vi "Efficiency Plot.vi"(0 "SMU 1 (Source)":refnum<k15>="4139_1", 1 "Voltage Steps":dbl[](array[numeric])=[8.5, 12.0, 24.0, 36.0, 48.0, 60.0], 5 "SMU 2 (Sink)":refnum<k15>="4139_2", 7 "Current Sweep Start":dbl format="%0.2f", 9 "Current Sweep End":dbl=-3.0 format="%0.2f", 11 "Error In":errorcluster, 12 "# Points":i32=50) -> (6 "Efficiency Plot":cluster{"current measurements":dbl[], dbl[]}[](graph)=[{"current measurements"=[0.0, 0.061224489795918366, 0.12244897959183673, 0.1836734693877551, 0.24489795918367346, 0.30612244897959184, 0.3673469387755102, 0.42857142857142855, 0.4897959183673469, 0.5510204081632653, 0.6122448979591837, 0.673469387755102, 0.7346938775510204, 0.7959183673469388, 0.8571428571428571, 0.9183673469387755, 0.9795918367346939, 1.0408163265306123, 1.1020408163265305, 1.163265306122449, 1.2244897959183674, 1.2857142857142858, 1.346938775510204, 1.4081632653061225, 1.469387755102041, 1.530612244897959, 1.5918367346938775, 1.653061224489796, 1.7142857142857142, 1.7755102040816326, 1.836734693877551, 1.8979591836734695, 1.9591836734693877, 2.020408163265306, 2.0816326530612246, 2.142857142857143, 2.204081632653061, 2.2653061224489797, 2.326530612244898, 2.3877551020408165, 2.4489795918367347, 2.510204081632653, 2.5714285714285716, 2.63265306122449, 2.693877551020408, 2.7551020408163267, 2.816326530612245, 2.877551020408163, 2.938775510204082, 3.0], [nan, inf, inf, inf, inf, inf, inf, inf, inf, inf, inf, inf, inf, inf, inf, inf, inf, inf, inf, inf, inf, inf, inf, inf, inf, inf, inf, inf, inf, inf, inf, inf, inf, inf, inf, inf, inf, inf, inf, inf, inf, inf, inf, inf, inf, inf, inf, inf, inf, inf]}, {"current measurements"=[0.0, 0.061224489795918366, 0.12244897959183673, 0.1836734693877551, 0.24489795918367346, 0.30612244897959184, 0.3673469387755102, 0.42857142857142855, 0.4897959183673469, 0.5510204081632653, 0.6122448979591837, 0.673469387755102, 0.7346938775510204, 0.7959183673469388, 0.8571428571428571, 0.9183673469387755, 0.9795918367346939, 1.0408163265306123, 1.1020408163265305, 1.163265306122449, 1.2244897959183674, 1.2857142857142858, 1.346938775510204, 1.4081632653061225, 1.469387755102041, 1.530612244897959, 1.5918367346938775, 1.653061224489796, 1.7142857142857142, 1.7755102040816326, 1.836734693877551, 1.8979591836734695, 1.9591836734693877, 2.020408163265306, 2.0816326530612246, 2.142857142857143, 2.204081632653061, 2.2653061224489797, 2.326530612244898, 2.3877551020408165, 2.4489795918367347, 2.510204081632653, 2.5714285714285716, 2.63265306122449, 2.693877551020408, 2.7551020408163267, 2.816326530612245, 2.877551020408163, 2.938775510204082, 3.0], [nan, inf, inf, inf, inf, inf, inf, inf, inf, inf, inf, inf, inf, inf, inf, inf, inf, inf, inf, inf, inf, inf, inf, inf, inf, inf, inf, inf, inf, inf, inf, inf, inf, inf, inf, inf, inf, inf, inf, inf, inf, inf, inf, inf, inf, inf, inf, inf, inf, inf]}, {"current measurements"=[0.0, 0.061224489795918366, 0.12244897959183673, 0.1836734693877551, 0.24489795918367346, 0.30612244897959184, 0.3673469387755102, 0.42857142857142855, 0.4897959183673469, 0.5510204081632653, 0.6122448979591837, 0.673469387755102, 0.7346938775510204, 0.7959183673469388, 0.8571428571428571, 0.9183673469387755, 0.9795918367346939, 1.0408163265306123, 1.1020408163265305, 1.163265306122449, 1.2244897959183674, 1.2857142857142858, 1.346938775510204, 1.4081632653061225, 1.469387755102041, 1.530612244897959, 1.5918367346938775, 1.653061224489796, 1.7142857142857142, 1.7755102040816326, 1.836734693877551, 1.8979591836734695, 1.9591836734693877, 2.020408163265306, 2.0816326530612246, 2.142857142857143, 2.204081632653061, 2.2653061224489797, 2.326530612244898, 2.3877551020408165, 2.4489795918367347, 2.510204081632653, 2.5714285714285716, 2.63265306122449, 2.693877551020408, 2.7551020408163267, 2.816326530612245, 2.877551020408163, 2.938775510204082, 3.0], [nan, inf, inf, inf, inf, inf, inf, inf, inf, inf, inf, inf, inf, inf, inf, inf, inf, inf, inf, inf, inf, inf, inf, inf, inf, inf, inf, inf, inf, inf, inf, inf, inf, inf, inf, inf, inf, inf, inf, inf, inf, inf, inf, inf, inf, inf, inf, inf, inf, inf]}, {"current measurements"=[0.0, 0.061224489795918366, 0.12244897959183673, 0.1836734693877551, 0.24489795918367346, 0.30612244897959184, 0.3673469387755102, 0.42857142857142855, 0.4897959183673469, 0.5510204081632653, 0.6122448979591837, 0.673469387755102, 0.7346938775510204, 0.7959183673469388, 0.8571428571428571, 0.9183673469387755, 0.9795918367346939, 1.0408163265306123, 1.1020408163265305, 1.163265306122449, 1.2244897959183674, 1.2857142857142858, 1.346938775510204, 1.4081632653061225, 1.469387755102041, 1.530612244897959, 1.5918367346938775, 1.653061224489796, 1.7142857142857142, 1.7755102040816326, 1.836734693877551, 1.8979591836734695, 1.9591836734693877, 2.020408163265306, 2.0816326530612246, 2.142857142857143, 2.204081632653061, 2.2653061224489797, 2.326530612244898, 2.3877551020408165, 2.4489795918367347, 2.510204081632653, 2.5714285714285716, 2.63265306122449, 2.693877551020408, 2.7551020408163267, 2.816326530612245, 2.877551020408163, 2.938775510204082, 3.0], [nan, inf, inf, inf, inf, inf, inf, inf, inf, inf, inf, inf, inf, inf, inf, inf, inf, inf, inf, inf, inf, inf, inf, inf, inf, inf, inf, inf, inf, inf, inf, inf, inf, inf, inf, inf, inf, inf, inf, inf, inf, inf, inf, inf, inf, inf, inf, inf, inf, inf]}, {"current measurements"=[0.0, 0.061224489795918366, 0.12244897959183673, 0.1836734693877551, 0.24489795918367346, 0.30612244897959184, 0.3673469387755102, 0.42857142857142855, 0.4897959183673469, 0.5510204081632653, 0.6122448979591837, 0.673469387755102, 0.7346938775510204, 0.7959183673469388, 0.8571428571428571, 0.9183673469387755, 0.9795918367346939, 1.0408163265306123, 1.1020408163265305, 1.163265306122449, 1.2244897959183674, 1.2857142857142858, 1.346938775510204, 1.4081632653061225, 1.469387755102041, 1.530612244897959, 1.5918367346938775, 1.653061224489796, 1.7142857142857142, 1.7755102040816326, 1.836734693877551, 1.8979591836734695, 1.9591836734693877, 2.020408163265306, 2.0816326530612246, 2.142857142857143, 2.204081632653061, 2.2653061224489797, 2.326530612244898, 2.3877551020408165, 2.4489795918367347, 2.510204081632653, 2.5714285714285716, 2.63265306122449, 2.693877551020408, 2.7551020408163267, 2.816326530612245, 2.877551020408163, 2.938775510204082, 3.0], [nan, inf, inf, inf, inf, inf, inf, inf, inf, inf, inf, inf, inf, inf, inf, inf, inf, inf, inf, inf, inf, inf, inf, inf, inf, inf, inf, inf, inf, inf, inf, inf, inf, inf, inf, inf, inf, inf, inf, inf, inf, inf, inf, inf, inf, inf, inf, inf, inf, inf]}, {"current measurements"=[0.0, 0.061224489795918366, 0.12244897959183673, 0.1836734693877551, 0.24489795918367346, 0.30612244897959184, 0.3673469387755102, 0.42857142857142855, 0.4897959183673469, 0.5510204081632653, 0.6122448979591837, 0.673469387755102, 0.7346938775510204, 0.7959183673469388, 0.8571428571428571, 0.9183673469387755, 0.9795918367346939, 1.0408163265306123, 1.1020408163265305, 1.163265306122449, 1.2244897959183674, 1.2857142857142858, 1.346938775510204, 1.4081632653061225, 1.469387755102041, 1.530612244897959, 1.5918367346938775, 1.653061224489796, 1.7142857142857142, 1.7755102040816326, 1.836734693877551, 1.8979591836734695, 1.9591836734693877, 2.020408163265306, 2.0816326530612246, 2.142857142857143, 2.204081632653061, 2.2653061224489797, 2.326530612244898, 2.3877551020408165, 2.4489795918367347, 2.510204081632653, 2.5714285714285716, 2.63265306122449, 2.693877551020408, 2.7551020408163267, 2.816326530612245, 2.877551020408163, 2.938775510204082, 3.0], [nan, inf, inf, inf, inf, inf, inf, inf, inf, inf, inf, inf, inf, inf, inf, inf, inf, inf, inf, inf, inf, inf, inf, inf, inf, inf, inf, inf, inf, inf, inf, inf, inf, inf, inf, inf, inf, inf, inf, inf, inf, inf, inf, inf, inf, inf, inf, inf, inf, inf]}], 15 "Error Out":errorcluster)   [LabVIEW 2014]
doc: "Demonstrates how to use triggers and events to synchronize multiple channels in Sequence source mode. Use this example to sequence multiple channels in lock-step."
uses:
  <instrlib>/niDCPower/nidcpower.llb/niDCPower Output Function.ctl
  <instrlib>/niDCPower/nidcpower.llb/niDCPower Source Mode.ctl
  <instrlib>/niDCPower/nidcpower.llb/niDCPower Sense.ctl
  <instrlib>/niDCPower/nidcpower.llb/niDCPower Sequence Attribute Type.ctl
  <instrlib>/niDCPower/nidcpower.llb/niDCPower Disable Source Trigger.vi
  <instrlib>/niDCPower/nidcpower.llb/niDCPower Configure Digital Edge Source Trigger.vi
  <instrlib>/niDCPower/nidcpower.llb/niDCPower Configure Digital Edge Measure Trigger.vi
panel:
  # "Sink"
  # "SOURCING OPERATION (SMU 1)\n1. Source Voltage Level and Fire Source Trigger Event \n2. Wait \"Delay\" Seconds\n3. Fire Source Complete Event\n3. Measure Current Immediately\n\nIV1, IV2, IV3...IV300 at V IN"
  # "SINKING OPERATION (SMU 2)\n1. Source Current Level (SMU1 Trigger)\n2. Wait \"Delay\" Seconds\n3. Measure Voltage (Using SMU1 Source Complete Event Trigger)\n\n\nIV1, IV2, IV3...IV300 at V OUT"
  # "Source"
  # "Iout = 0 to 3 A"
  # "Vin = 8 to 60 V"
  # "Vout = 5 V"
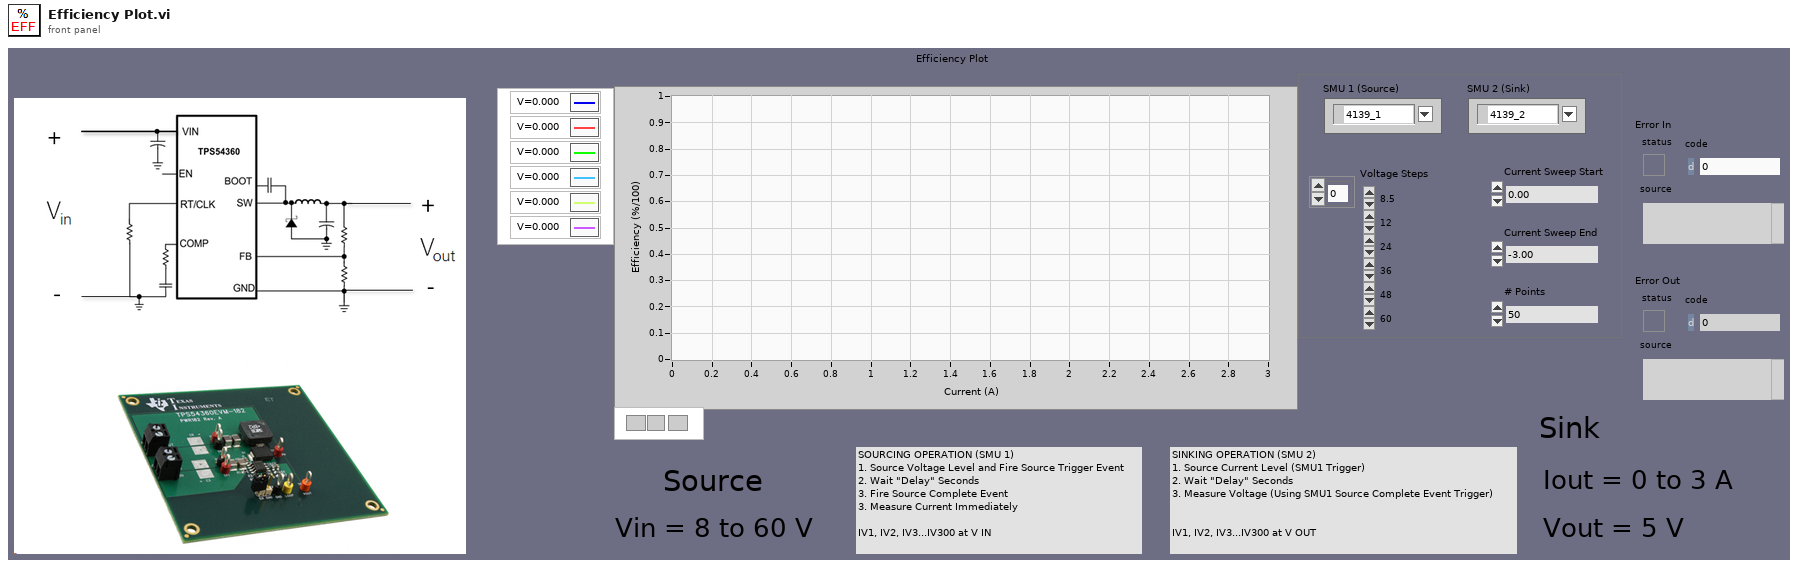
[diagram p1: front panel]
types:
  T1 = typedef "niDCPower Sequence Attribute Type.ctl" = i32
  T2 = typedef "niDCPower Sense.ctl" = i32
  T3 = typedef "niDCPower Source Mode.ctl" = i32
  T4 = typedef "niDCPower Output Function.ctl" = i32
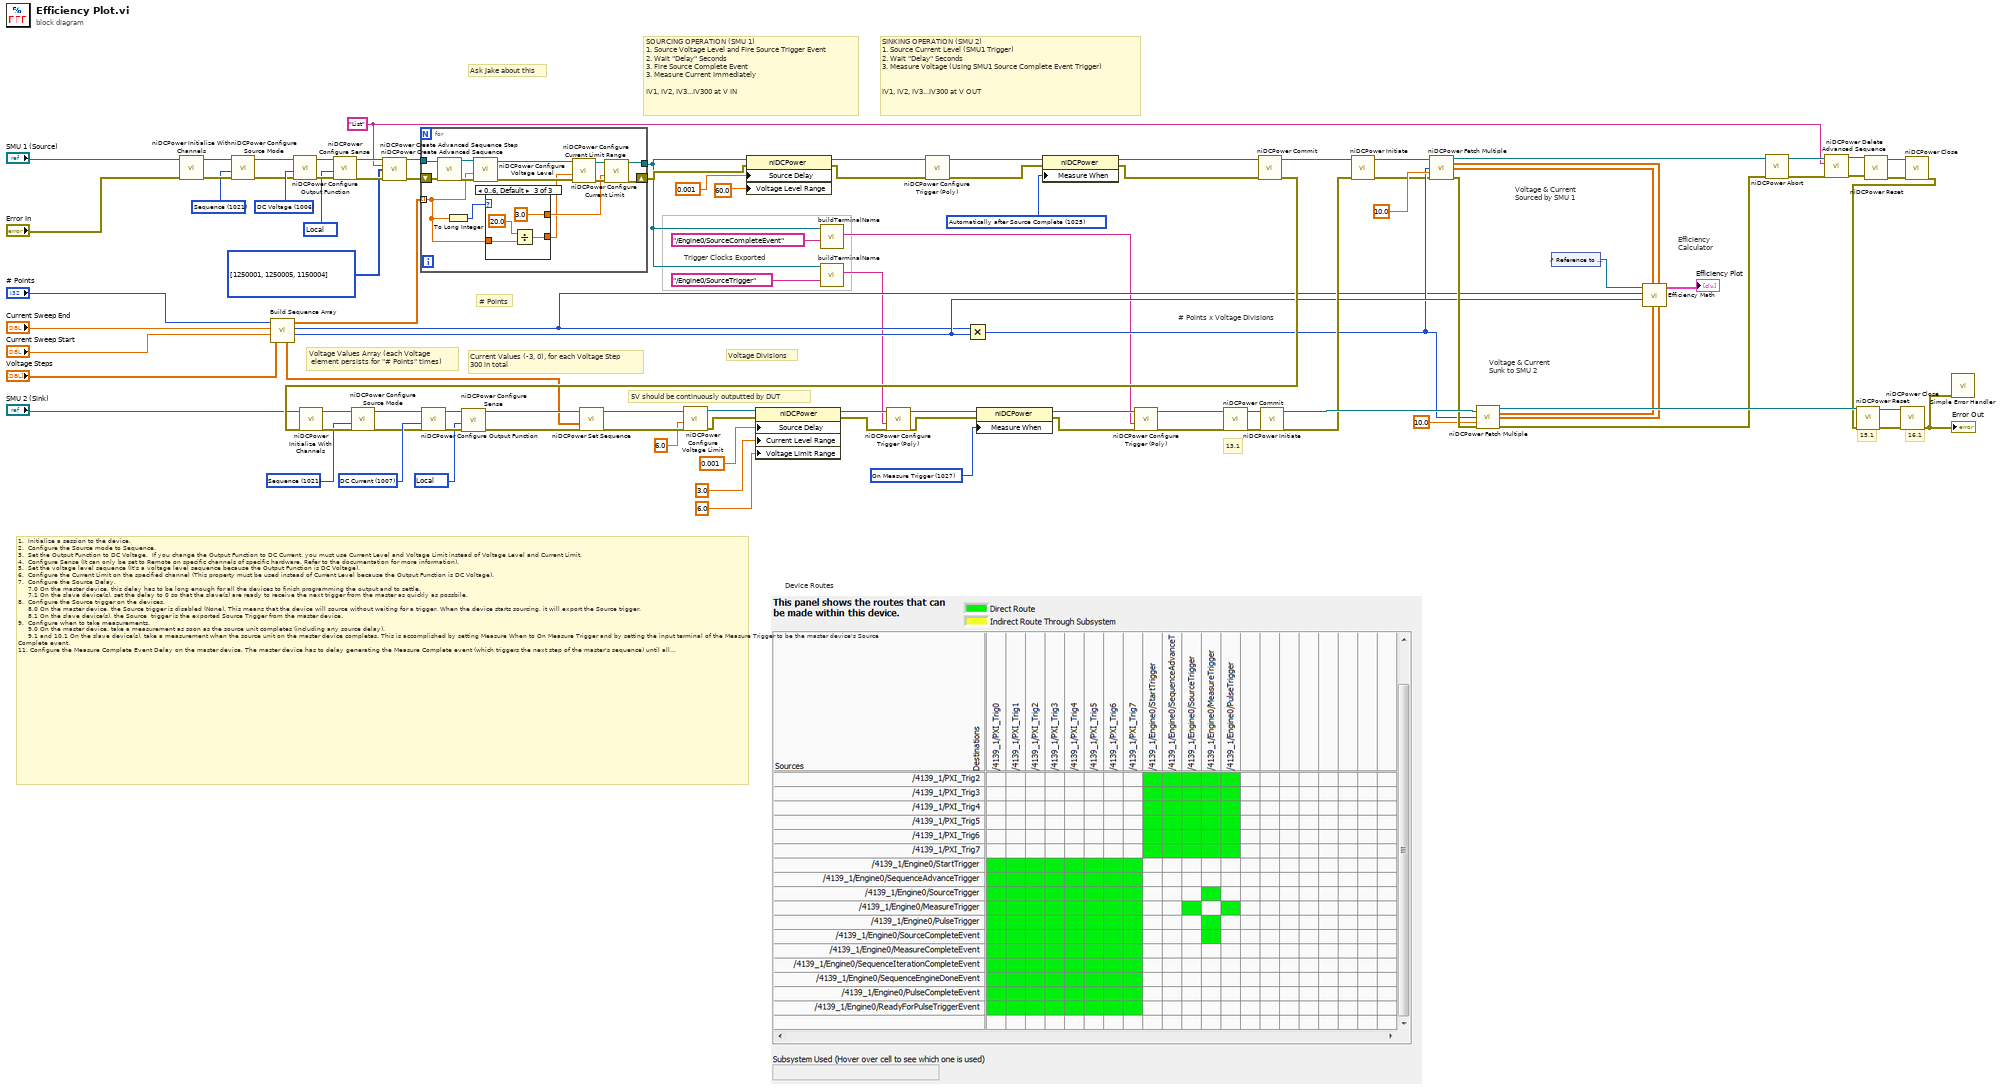
[diagram p0: block diagram]
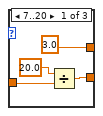
[diagram p2: hidden frame]
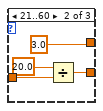
[diagram p3: hidden frame]
diagram:
  w2 = "List" ("list name")
  w18 = T1[] [1250001, 1250005, 1150004] items=["Voltage Pole-Zero Ratio"=1150069, "Voltage Compensation Frequency"=1150068, "Voltage Gain Bandwidth"=1150067, "Transient Response"=1150062, "Output Resistance"=1150061, "Output Connected"=1150060, "Output Enabled"=1250006, "Output Function"=1150008, "Source Delay"=1150051, "Aperture Time Units"=1150059, "Aperture Time"=1150058, "Voltage Limit Range"=1150012, "Voltage Limit"=1150010, "Current Level Range"=1150011, "Current Level"=1150009, "Current Limit Range"=1150004, "Current Limit"=1250005, "Voltage Level Range"=1150005, "Voltage Level"=1250001]
  w52 = T2 1008 items=["Local"=1008, "Remote"=1009] ("sense")
  w53 = T2 1008 items=["Local"=1008, "Remote"=1009] ("sense")
  w65 = 1027 items=["Automatically after Source Complete"=1025, "On Demand"=1026, "On Measure Trigger"=1027] ("Measurement:Advanced:Measure When")
  w66 = T3 1021 items=["Single Point"=1020, "Sequence"=1021] ("source mode")
  w77 = T4 1007 items=["DC Voltage"=1006, "DC Current"=1007] ("output function")
  w86 = 1025 items=["Automatically after Source Complete"=1025, "On Demand"=1026, "On Measure Trigger"=1027] ("Measurement:Advanced:Measure When")
  w87 = T3 1021 items=["Single Point"=1020, "Sequence"=1021] ("source mode")
  w94 = T4 1006 items=["DC Voltage"=1006, "DC Current"=1007] ("output function")
  # "Trigger Clocks Exported"
  # "Device Routes"
  # "Efficiency\nCalculator"
  # "Voltage & Current \nSourced by SMU 1"
  # "Voltage & Current \nSunk to SMU 2"
  # "# Points x Voltage Divisions"
  # "Ask Jake about this"
  # "SINKING OPERATION (SMU 2)\n1. Source Current Level (SMU1 Trigger)\n2. Wait \"Delay\" Seconds\n3. Measure Voltage (Using SMU1 Source Complete Event Trigger)\n\n\nIV1, IV2, IV3...IV300 at V OUT"
  # "SOURCING OPERATION (SMU 1)\n1. Source Voltage Level and Fire Source Trigger Event \n2. Wait \"Delay\" Seconds\n3. Fire Source Complete Event\n3. Measure Current Immediately\n\nIV1, IV2, IV3...IV300 at V IN"
  # "Voltage Divisions"
  # "# Points"
  # "5V should be continuously outputted by DUT"
  # "Voltage Values Array (each Voltage\n element persists for \"# Points\" times)"
  # "Current Values (-3, 0), for each Voltage Step\n300 in total"
  # "16.1"
  # "15.1"
  # "13.1"
  # "1.  Initialize a session to the device.\n2.  Configure the Source mode to Sequence.\n3.  Set the Output Function to DC Voltage.  If you change the Output Function to DC Current, you must use Current Level and Voltage Limit instead of Voltage Level and Current Limit.\n4.  Configure Sense (It can only be set to Remote on specific channels of specific hardware. Refer to the documentation for more information).\n5.  Set the voltage level sequence (It's a voltage level sequence because the Output Function is DC Voltage).\n6.  Configure the Current Limit on the specified channel (This property must be used instead of Current Level because the Output Function is DC Voltage).\n7.  Configure the Source Delay.\n     7.0 On the master device, this delay has to be long enough for all the devices to finish programming the output and to settle.\n     7.1 On the slave device(s), set the delay to 0 so that the slave(s) are ready to receive the next trigger from the master as quickly as possbile.\n8.  Configure the Source trigger on the devices.\n     8.0 On the master device, the Source trigger is disabled (None). This means that the device will source without waiting for a trigger. When the device starts sourcing, it will export the Source trigger.\n     8.1 On the slave device(s), the Source  trigger is the exported Source Trigger from the master device.\n9.  Configure when to take measurements.\n     9.0 On the master device, take a measurement as soon as the source unit completes (including any source delay).\n     9.1 and 10.1 On the slave device(s), take a measurement when the source unit on the master device completes. This is accomplished by setting Measure When to On Measure Trigger and by setting the input terminal of the Measure Trigger to be the master device's Source Complete event.\n11. Configure the Measure Complete Event Delay on the master device. The master device has to delay generating the Measure Complete event (which triggers the next step of the master's sequence) until all slave device(s) have completed taking measurements. The amount of time a slave takes to measure can vary based on its configuration and model.\n12. Commit the settings to the device so that the driver establishes all the routing required for the configured triggers and events."
  n1 = call <instrlib>:"niDCPower Initialize With Channels.vi"("error in (no error)"="Error In", "resource name"="SMU 1 (Source)") -> ("error out"=w91:errorcluster, "instrument handle out"=w88:refnum<k15>)  [unwired: 2 in, 6 out]
  n2 = call <instrlib>:"niDCPower Configure Source Mode.vi"("error in (no error)"=w91, "source mode"=w87, "instrument handle"=w88) -> ("error out"=w90:errorcluster, "instrument handle out"=w89:refnum<k15>)  [unwired: 7 out]
  n3 = call "Build Sequence Array.vi"("Voltage Steps"="Voltage Steps", "Current Sweep Start"="Current Sweep Start", "Current Sweep End"="Current Sweep End", "# Points"="# Points") -> ("# Voltage Divisions"=w33:i32, "# of Points"=w28:i32, "To SMU 1 (Source)"=w27:dbl[], "To SMU 2 (Sink)"=w26:dbl[])  [unwired: 4 in]
  n4 = call <instrlib>:"niDCPower Configure Output Function.vi"("error in (no error)"=w90, "output function"=w94, "instrument handle"=w89) -> ("error out"=w96:errorcluster, "instrument handle out"=w95:refnum<k15>)  [unwired: 1 in, 6 out]
  n5 = call <instrlib>:"niDCPower Configure Sense.vi"("error in (no error)"=w96, "sense"=w52, "instrument handle"=w95) -> ("error out"=w21:errorcluster, "instrument handle out"=w22:refnum<k15>)  [unwired: 1 in, 6 out]
  n6 = call <instrlib>:"niDCPower Create Advanced Sequence.vi"("instrument handle"=w22, "sequence name"=w2, "advanced sequence properties"=w18, "error in (no error)"=w21) -> ("instrument handle out"=w19:refnum<k15>, "error out"=w20:errorcluster)  [unwired: 10 in]
  n7 = for {
    tunnel: w19 -> [w106]
    tunnel: [w110] -> w15
    shift-right: [w109] -> w34
    shift-left: w20 -> [w103]
    tunnel: w27 -> [w102] mode=indexing
    n8 = call <instrlib>:"niDCPower Create Advanced Sequence Step.vi"("error in (no error)"=w103, "instrument handle"=w106) -> ("error out"=w104:errorcluster, "instrument handle out"=w105:refnum<k15>)  [unwired: 8 in]
    n9 = To Long Integer(number=w102) -> (32bit integer=w101:i32)
    n10 = call <instrlib>:"niDCPower Configure Voltage Level.vi"("error in (no error)"=w104, "voltage level"=w102, "instrument handle"=w105) -> ("error out"=w114:errorcluster, "instrument handle out"=w113:refnum<k15>)  [unwired: 7 in]
    n11 = case shown="0..6, Default" w101 {
      tunnel: [3.0 3.0 3.0] -> w108
      tunnel: w102 -> [w116 w119 w125]
      tunnel: [w115 w121 w123] -> w107
      frame 7..20 {
        n12 = Divide(x=20.0, y=w116) -> (x/y=w115:dbl)
      }
      frame 21..60 {
        n13 = Divide(x=20.0, y=w119) -> (x/y=w121:dbl)
      }
      frame 0..6, Default {
        n14 = Divide(x=20.0, y=w125) -> (x/y=w123:dbl)
      }
    }
    n15 = call <instrlib>:"niDCPower Configure Current Limit.vi"("error in (no error)"=w114, "current limit"=w107, "instrument handle"=w113) -> ("error out"=w111:errorcluster, "instrument handle out"=w112:refnum<k15>)  [unwired: 2 in, 5 out]
    n16 = call <instrlib>:"niDCPower Configure Current Limit Range.vi"("error in (no error)"=w111, "current limit range"=w108, "instrument handle"=w112) -> ("error out"=w109:errorcluster, "instrument handle out"=w110:refnum<k15>)  [unwired: 7 in]
  }
  n17 = property class="niDCPower"(reference=w15, error in=w34, "Source Delay"=0.001 ("Source:Advanced:Source Delay"), "Voltage Level Range"=60.0 ("Source:Advanced:Source Delay")) -> (reference out=w31:refnum<k15>, error out=w30:errorcluster)
  n18 = call "buildTerminalName.vi"("Local Terminal Name"="/Engine0/SourceCompleteEvent", "session handle"=w15) -> ("Fully Qualified Terminal Name"=w16:string)  [unwired: 7 in, 2 out]
  n19 = call "buildTerminalName.vi"("Local Terminal Name"="/Engine0/SourceTrigger", "session handle"=w15) -> ("Fully Qualified Terminal Name"=w1:string)  [unwired: 7 in, 2 out]
  n20 = call-poly <instrlib>:"niDCPower Configure Trigger (Poly).vi"("error in (no error)"=w30, "instrument handle"=w31) -> ("error out"=w92:errorcluster, "instrument handle out"=w93:refnum<k15>)  [unwired: 1 in, 7 out]
  n21 = Multiply(x=w28, y=w33) -> (x*y=w32:i32)
  n22 = property class="niDCPower"(reference=w93, error in=w92, "Measure When"=w86) -> (reference out=w81:refnum<k15>, error out=w80:errorcluster)
  n23 = call <instrlib>:"niDCPower Commit.vi"("error in (no error)"=w80, "instrument handle"=w81) -> ("error out"=w83:errorcluster, "instrument handle out"=w84:refnum<k15>)  [unwired: 8 out]
  n24 = call <instrlib>:"niDCPower Initialize With Channels.vi"("error in (no error)"=w83, "resource name"="SMU 2 (Sink)") -> ("error out"=w70:errorcluster, "instrument handle out"=w67:refnum<k15>)  [unwired: 2 in, 6 out]
  n25 = call <instrlib>:"niDCPower Configure Source Mode.vi"("error in (no error)"=w70, "source mode"=w66, "instrument handle"=w67) -> ("error out"=w69:errorcluster, "instrument handle out"=w68:refnum<k15>)  [unwired: 7 out]
  n26 = call <instrlib>:"niDCPower Configure Output Function.vi"("error in (no error)"=w69, "output function"=w77, "instrument handle"=w68) -> ("error out"=w79:errorcluster, "instrument handle out"=w78:refnum<k15>)  [unwired: 1 in, 6 out]
  n27 = call <instrlib>:"niDCPower Configure Sense.vi"("error in (no error)"=w79, "sense"=w53, "instrument handle"=w78) -> ("error out"=w75:errorcluster, "instrument handle out"=w76:refnum<k15>)  [unwired: 1 in, 6 out]
  n28 = call <instrlib>:"niDCPower Set Sequence.vi"("error in (no error)"=w75, "values"=w26, "instrument handle"=w76) -> ("error out"=w61:errorcluster, "instrument handle out"=w62:refnum<k15>)  [unwired: 2 in, 5 out]
  n29 = call <instrlib>:"niDCPower Configure Voltage Limit.vi"("error in (no error)"=w61, "voltage limit"=6.0, "instrument handle"=w62) -> ("error out"=w60:errorcluster, "instrument handle out"=w59:refnum<k15>)  [unwired: 7 in]
  n30 = property class="niDCPower"(reference=w59, error in=w60, "Source Delay"=0.001 ("Source:Advanced:Source Delay"), "Current Level Range"=3.0 ("Source:Advanced:Source Delay"), "Voltage Limit Range"=6.0 ("Source:Advanced:Source Delay")) -> (reference out=w63:refnum<k15>, error out=w64:errorcluster)
  n31 = call-poly <instrlib>:"niDCPower Configure Trigger (Poly).vi"("error in (no error)"=w64, "input terminal"=w1, "instrument handle"=w63) -> ("error out"=w73:errorcluster, "instrument handle out"=w74:refnum<k15>)  [unwired: 1 in, 6 out]
  n32 = property class="niDCPower"(reference=w74, error in=w73, "Measure When"=w65) -> (reference out=w71:refnum<k15>, error out=w72:errorcluster)
  n33 = call-poly <instrlib>:"niDCPower Configure Trigger (Poly).vi"("error in (no error)"=w72, "input terminal"=w16, "instrument handle"=w71) -> ("error out"=w50:errorcluster, "instrument handle out"=w51:refnum<k15>)  [unwired: 1 in, 6 out]
  n34 = call <instrlib>:"niDCPower Commit.vi"("error in (no error)"=w50, "instrument handle"=w51) -> ("error out"=w98:errorcluster, "instrument handle out"=w99:refnum<k15>)  [unwired: 8 out]
  n35 = call <instrlib>:"niDCPower Initiate.vi"("error in (no error)"=w98, "instrument handle"=w99) -> ("error out"=w85:errorcluster, "instrument handle out"=w100:refnum<k15>)  [unwired: 8 out]
  n36 = call <instrlib>:"niDCPower Initiate.vi"("error in (no error)"=w85, "instrument handle"=w84) -> ("error out"=w25:errorcluster, "instrument handle out"=w24:refnum<k15>)  [unwired: 8 out]
  n37 = call <instrlib>:"niDCPower Fetch Multiple.vi"("instrument handle"=w24, "count (1)"=w32, "timeout (sec)"=10.0, "error in (no error)"=w25) -> ("instrument handle out"=w8:refnum<k15>, "voltage measurements"=w42:dbl[], "current measurements"=w43:dbl[], "error out"=w82:errorcluster)  [unwired: 1 in, 7 out]
  n38 = call <instrlib>:"niDCPower Fetch Multiple.vi"("instrument handle"=w100, "count (1)"=w32, "timeout (sec)"=10.0, "error in (no error)"=w82) -> ("instrument handle out"=w97:refnum<k15>, "voltage measurements"=w44:dbl[], "current measurements"=w40:dbl[], "error out"=w9:errorcluster)  [unwired: 1 in, 7 out]
  n39 = control-ref of="Reference to XY Graph"() -> (w13:refnum<vi>)
  n40 = call "Efficiency Math.vi"("SMU 2 Current Measurements"=w40, "SMU 1 Voltage Measurements"=w42, "SMU 2 Voltage Measurements"=w44, "SMU 1 Current Measurements"=w43, "# Voltage Divisions"=w33, "# Points"=w28, "XYGraph in"=w13) -> ("Array"=→"Efficiency Plot":cluster{"Array":dbl[], "Array":dbl[]}[])  [unwired: 4 in]
  n41 = call <instrlib>:"niDCPower Abort.vi"("error in (no error)"=w9, "instrument handle"=w8) -> ("error out"=w4:errorcluster, "instrument handle out"=w7:refnum<k15>)  [unwired: 8 in]
  n42 = call <instrlib>:"niDCPower Delete Advanced Sequence.vi"("error in (no error)"=w4, "sequence name"=w2, "instrument handle"=w7) -> ("error out"=w5:errorcluster, "instrument handle out"=w6:refnum<k15>)  [unwired: 7 in]
  n43 = call <instrlib>:"niDCPower Reset.vi"("error in (no error)"=w5, "instrument handle"=w6) -> ("error out"=w12:errorcluster, "instrument handle out"=w11:refnum<k15>)  [unwired: 1 in, 7 out]
  n44 = call <instrlib>:"niDCPower Close.vi"("error in (no error)"=w12, "instrument handle"=w11) -> ("error out"=w3:errorcluster)  [unwired: 9 out]
  n45 = call <instrlib>:"niDCPower Reset.vi"("error in (no error)"=w3, "instrument handle"=w97) -> ("error out"=w58:errorcluster, "instrument handle out"=w57:refnum<k15>)  [unwired: 1 in, 7 out]
  n46 = call <instrlib>:"niDCPower Close.vi"("error in (no error)"=w58, "instrument handle"=w57) -> ("error out"=w10:errorcluster)  [unwired: 9 out]
  "Error Out" <- w10
  n47 = call <vilib>:"Simple Error Handler.vi"("error in (no error)"=w10) -> ()  [unwired: 4 in, 5 out]
